vi "FPGA_Qudi_Scan_trigger_camera_synchro_laser_lines_v2.vi"(3 "N Z positions":i32) -> ()   [LabVIEW 2015]
uses:
  <vilib>/eio/EIONode/EIONode.xnode
  <vilib>/rvi/eio/common/nirviEmuTemplateMethod_errors.vi
panel:
  out "Images acquired":i32
  in  "Laser lines":i32[](array[numeric])=[0, 0, 0, 0, 0]
  in  "Laser power":i16[](array[numeric])=[0, 0, 0, 0, 0]
  in  "N laser lines":i32
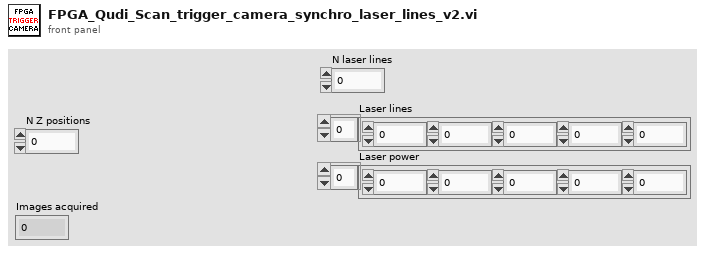
[diagram p1: front panel]
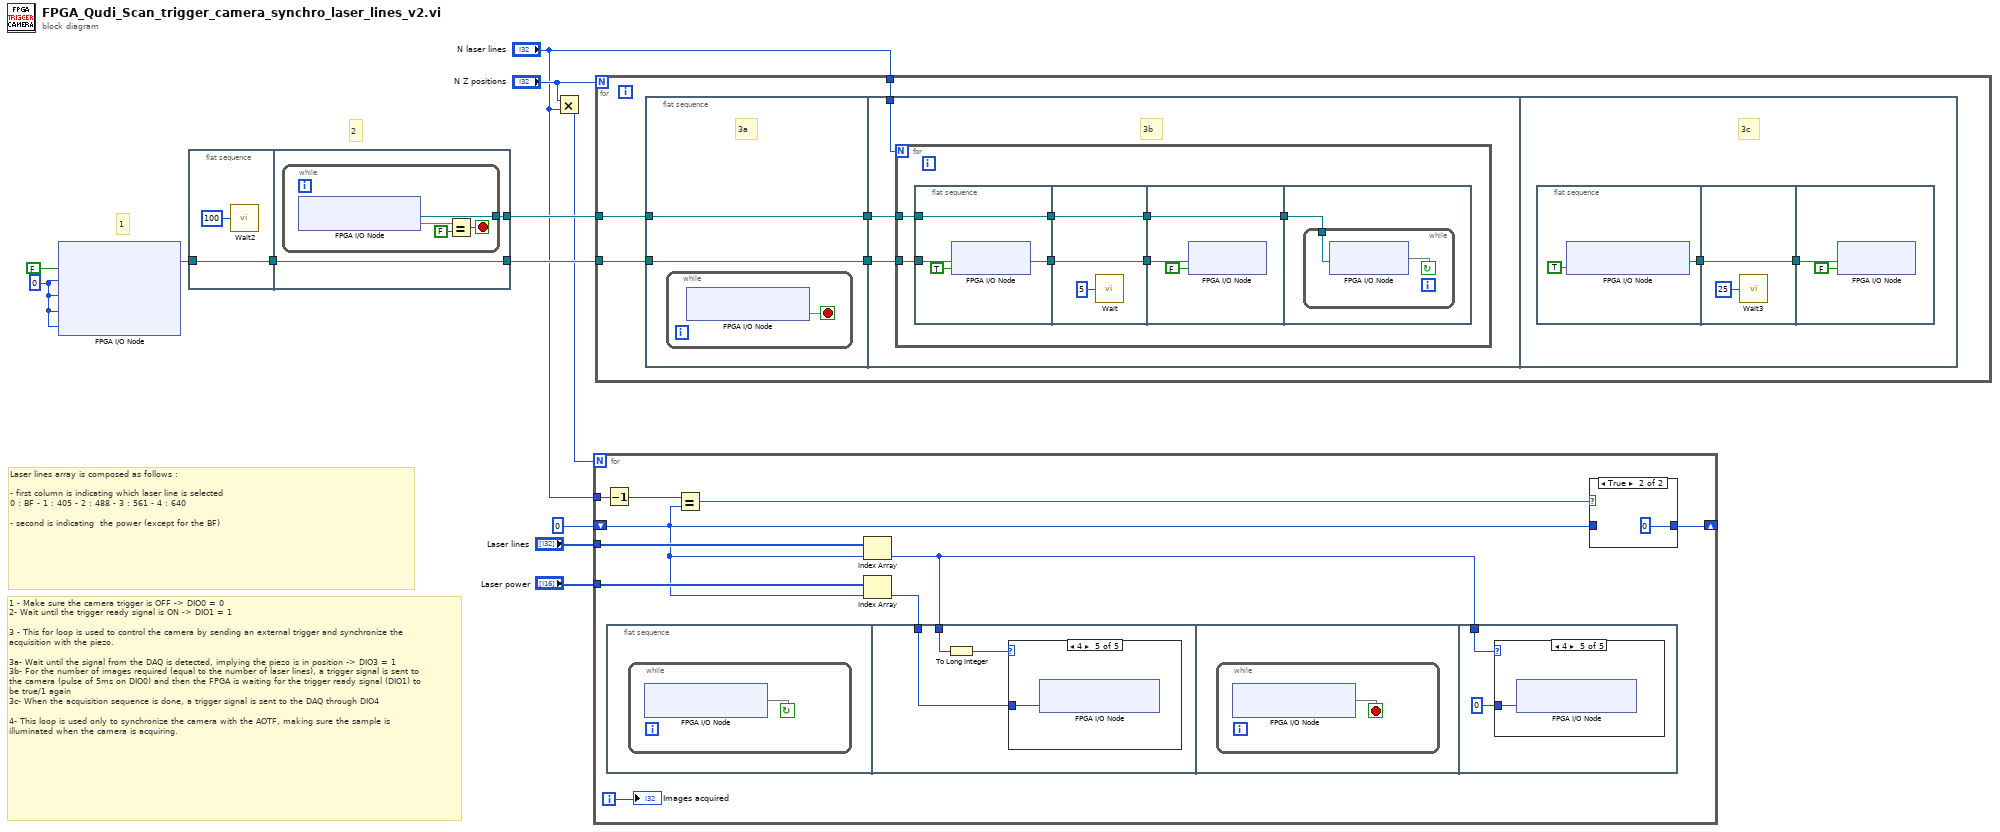
[diagram p0: block diagram]
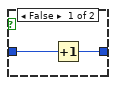
[diagram p2: hidden frame]
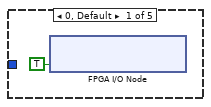
[diagram p3: hidden frame]
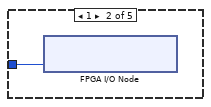
[diagram p4: hidden frame]
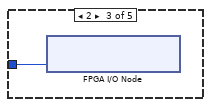
[diagram p5: hidden frame]
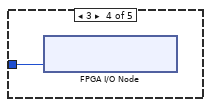
[diagram p6: hidden frame]
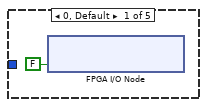
[diagram p7: hidden frame]
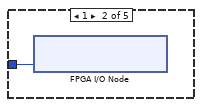
[diagram p8: hidden frame]
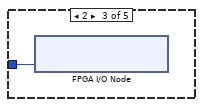
[diagram p9: hidden frame]
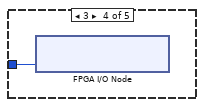
[diagram p10: hidden frame]
diagram:
  w1 = i16 0 ("Connector0/AO0")
  # "2"
  # "1"
  # "1 - Make sure the camera trigger is OFF -> DIO0 = 0\n2- Wait until the trigger ready signal is ON -> DIO1 = 1\n\n3 - This for loop is used to control the camera by sending an external trigger and synchronize the acquisition with the piezo.\n\n3a- Wait until the signal from the DAQ is detected, implying the piezo is in position -> DIO3 = 1 \n3b- For the number of images required (equal to the number of laser lines), a trigger signal is sent to the camera (pulse of 5ms on DIO0) and then the FPGA is waiting for the trigger ready signal (DIO1) to be true/1 again\n3c- When the acquisition sequence is done, a trigger signal is sent to the DAQ through DIO4\n\n4- This loop is used only to synchronize the camera with the AOTF, making sure the sample is illuminated when the camera is acquiring."
  # "Laser lines array is composed as follows :\n\n- first column is indicating which laser line is selected \n0 : BF - 1 : 405 - 2 : 488 - 3 : 561 - 4 : 640\n\n- second is indicating  the power (except for the BF)"
  n1 = xnode "FPGA I/O Node"("Connector0/DIO0"=FALSE, "Connector0/AO0"=w1, "Connector0/AO1"=w1, "Connector0/AO2"=w1, "Connector0/AO3"=w1) -> ("FPGA I/O Out"=w11:refnum<k21>)  [unwired: 5 in, 4 out]
  n2 = flat-sequence {
    tunnel: w11 -> [w14]
    tunnel: [w14] -> w10
    tunnel: w10 -> [w16]
    tunnel: [w16] -> w9
    tunnel: [w15] -> w8
    frame #0 {
      n3 = call "Wait2"("Count(uSec)"=u32 100 ("Count(mSec)")) -> ()  [unwired: 1 out]
    }
    frame #1 {
      n4 = while {
        tunnel: [w20] -> w15
        stop <- w17 stop-if-true
        n5 = xnode "FPGA I/O Node"() -> ("Connector0/DIO1"=w19, "FPGA I/O Out"=w20:refnum<k21>)  [unwired: 1 in]
        n6 = Equal?(x=w19, y=FALSE) -> (x = y?=w17:bool)
      }
    }
  }
  n7 = Multiply(x="N Z positions", y="N laser lines") -> (x*y=w3:i32)
  n8 = for {
    N: w3 -> [_]
    shift-right: [w28] -> _
    shift-left: 0 -> [w25]
    tunnel: "Laser lines" -> [w27]
    tunnel: "Laser power" -> [w26]
    tunnel: "N laser lines" -> [w23]
    i -> [w21]
    n9 = Decrement(x=w23) -> (x-1=w22:i32)
    n10 = flat-sequence {
      tunnel: w30 -> [w36]
      tunnel: w24 -> [w35]
      tunnel: w30 -> [w44]
      frame #0 {
        n11 = while {
          stop <- w34 continue-if-true
          n12 = xnode "FPGA I/O Node"() -> ("Connector0/DIO2"=w34)  [unwired: 1 in, 1 out]
        }
      }
      frame #1 {
        n13 = To Long Integer(number=w36) -> (32bit integer=w37:i32)
        n14 = case shown="4" w37 {
          tunnel: w35 -> [_ w39 w40 w41 w42]
          frame 0, Default {
            n15 = xnode "FPGA I/O Node"("Connector0/DIO5"=TRUE) -> ()  [unwired: 1 in, 1 out]
          }
          frame 1 {
            n16 = xnode "FPGA I/O Node"("Connector0/AO2"=w39) -> ()  [unwired: 1 in, 1 out]
          }
          frame 2 {
            n17 = xnode "FPGA I/O Node"("Connector0/AO3"=w40) -> ()  [unwired: 1 in, 1 out]
          }
          frame 3 {
            n18 = xnode "FPGA I/O Node"("Connector0/AO0"=w41) -> ()  [unwired: 1 in, 1 out]
          }
          frame 4 {
            n19 = xnode "FPGA I/O Node"("Connector0/AO1"=w42) -> ()  [unwired: 1 in, 1 out]
          }
        }
      }
      frame #2 {
        n20 = while {
          stop <- w43 stop-if-true
          n21 = xnode "FPGA I/O Node"() -> ("Connector0/DIO2"=w43)  [unwired: 1 in, 1 out]
        }
      }
      frame #3 {
        n22 = case shown="4" w44 {
          tunnel: i16 0 -> [_ w47 w48 w49 w50]
          frame 0, Default {
            n23 = xnode "FPGA I/O Node"("Connector0/DIO5"=FALSE) -> ()  [unwired: 1 in, 1 out]
          }
          frame 1 {
            n24 = xnode "FPGA I/O Node"("Connector0/AO2"=w47) -> ()  [unwired: 1 in, 1 out]
          }
          frame 2 {
            n25 = xnode "FPGA I/O Node"("Connector0/AO3"=w48) -> ()  [unwired: 1 in, 1 out]
          }
          frame 3 {
            n26 = xnode "FPGA I/O Node"("Connector0/AO0"=w49) -> ()  [unwired: 1 in, 1 out]
          }
          frame 4 {
            n27 = xnode "FPGA I/O Node"("Connector0/AO1"=w50) -> ()  [unwired: 1 in, 1 out]
          }
        }
      }
    }
    n28 = Equal?(x=w22, y=w25) -> (x = y?=w29:bool)
    n29 = Index Array(array=w27, index=w25) -> (element=w30:i32)
    n30 = Index Array(array=w26, index=w25) -> (element=w24:i16)
    n31 = case shown="True" w29 {
      tunnel: w25 -> [w32 _]
      tunnel: [w31 0] -> w28
      frame False {
        n32 = Increment(x=w32) -> (x+1=w31:i32)
      }
      frame True {
      }
    }
    "Images acquired" <- w21
  }
  n33 = for {
    N: "N Z positions" -> [_]
    tunnel: w9 -> [w54]
    tunnel: w8 -> [w55]
    tunnel: "N laser lines" -> [w51]
    n34 = flat-sequence {
      tunnel: w54 -> [w56]
      tunnel: w55 -> [w57]
      tunnel: [w57] -> w53
      tunnel: [w56] -> w52
      tunnel: w53 -> [w61]
      tunnel: w52 -> [w60]
      tunnel: w51 -> [w59]
      frame #0 {
        # "3a"
        n35 = while {
          stop <- w58 stop-if-true
          n36 = xnode "FPGA I/O Node"() -> ("Connector0/DIO3"=w58)  [unwired: 1 in, 1 out]
        }
      }
      frame #1 {
        # "3b"
        n37 = for {
          N: w59 -> [_]
          tunnel: w61 -> [w63]
          tunnel: w60 -> [w62]
          n38 = flat-sequence {
            tunnel: [w71] -> w68
            tunnel: [w69] -> w67
            tunnel: w62 -> [w70]
            tunnel: w63 -> [w69]
            tunnel: w68 -> [w74]
            tunnel: [w74] -> w66
            tunnel: [w73] -> w65
            tunnel: w67 -> [w73]
            tunnel: w66 -> [w77]
            tunnel: [w76] -> w64
            tunnel: w65 -> [w76]
            tunnel: w64 -> [w79]
            frame #0 {
              n39 = xnode "FPGA I/O Node"("I/O Item"=TRUE ("Connector0/DIO0"), "FPGA I/O In"=w70) -> ("FPGA I/O Out"=w71:refnum<k21>)
            }
            frame #1 {
              n40 = call "Wait"("Count(mSec)"=u32 5) -> ()  [unwired: 1 out]
            }
            frame #2 {
              n41 = xnode "FPGA I/O Node"("I/O Item"=FALSE ("Connector0/DIO0"), "FPGA I/O In"=w77) -> ()  [unwired: 1 out]
            }
            frame #3 {
              n42 = while {
                tunnel: w79 -> [w81]
                stop <- w80 continue-if-true
                n43 = xnode "FPGA I/O Node"("FPGA I/O In"=w81) -> ("I/O Item"=w80)  [unwired: 1 out]
              }
            }
          }
        }
      }
      frame #2 {
        # "3c"
        n44 = flat-sequence {
          tunnel: [w85] -> w83
          tunnel: w83 -> [w86]
          tunnel: [w86] -> w82
          tunnel: w82 -> [w88]
          frame #0 {
            n45 = xnode "FPGA I/O Node"("Connector0/DIO4"=TRUE) -> ("FPGA I/O Out"=w85:refnum<k21>)  [unwired: 1 in]
          }
          frame #1 {
            n46 = call "Wait3"("Count(mSec)"=u32 25) -> ()  [unwired: 1 out]
          }
          frame #2 {
            n47 = xnode "FPGA I/O Node"("I/O Item"=FALSE ("Connector0/DIO0"), "FPGA I/O In"=w88) -> ()  [unwired: 1 out]
          }
        }
      }
    }
  }
